vi "startIVSweepAndWait.vi"(8 "error in (no error)":errorcluster, 10 "setSweepConfiguration":variant, 11 "Instrument.LockinAPI in":refnum<class "Instrument.LockinAPI.lvclass">) -> (0 "error out":errorcluster, 3 "Instrument.LockinAPI out":refnum<class "Instrument.LockinAPI.lvclass">)   [LabVIEW 2019, in "Instrument.LockinAPI.lvclass"]
uses:
  Instrument.LockinAPI.lvclass
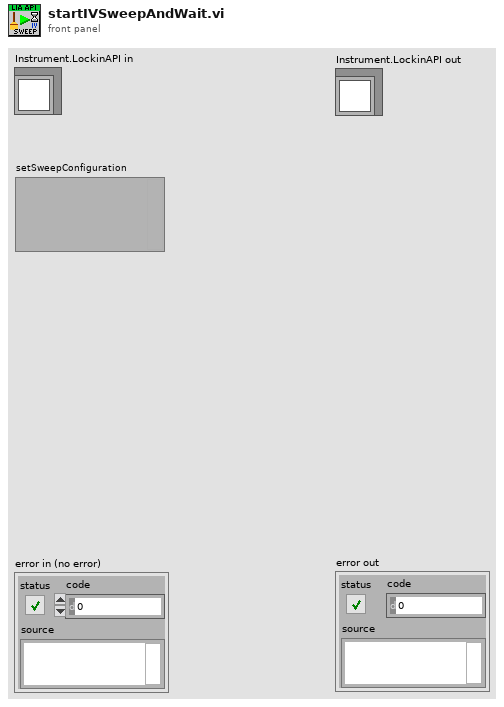
[diagram p1: front panel]
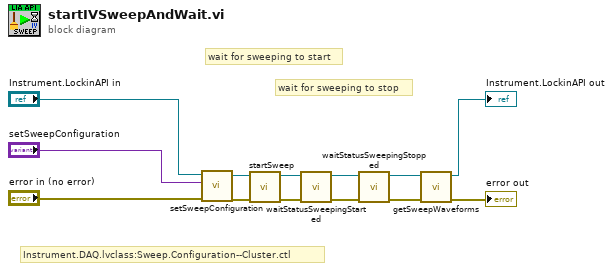
[diagram p0: block diagram]
diagram:
  # "Instrument.DAQ.lvclass:Sweep.Configuration--Cluster.ctl"
  # "wait for sweeping to stop"
  # "wait for sweeping to start"
  n1 = call-dynamic "setSweepConfiguration.vi"("error in (no error)"="error in (no error)", "setSweepConfiguration"="setSweepConfiguration", "Instrument.LockinAPI in"="Instrument.LockinAPI in") -> ("error out"=w9:errorcluster, "Instrument.LockinAPI out"=w10:refnum<class "Instrument.LockinAPI.lvclass">)  [unwired: 7 in]
  n2 = call "startSweep.vi"("error in (no error)"=w9, "Instrument.LockinAPI in"=w10) -> ("error out"=w5:errorcluster, "Instrument.LockinAPI out"=w6:refnum<class "Instrument.LockinAPI.lvclass">)  [unwired: 8 in]
  n3 = call "waitStatusSweepingStarted.vi"("error in (no error)"=w5, "Instrument.LockinAPI in"=w6) -> ("error out"=w4:errorcluster, "Instrument.LockinAPI out"=w7:refnum<class "Instrument.LockinAPI.lvclass">)  [unwired: 8 in]
  n4 = call "waitStatusSweepingStopped.vi"("error in (no error)"=w4, "Instrument.LockinAPI in"=w7) -> ("error out"=w3:errorcluster, "Instrument.LockinAPI out"=w2:refnum<class "Instrument.LockinAPI.lvclass">)  [unwired: 8 in]
  n5 = call-dynamic "getSweepWaveforms.vi"("error in (no error)"=w3, "Instrument.LockinAPI in"=w2) -> ("error out"=→"error out":errorcluster, "Instrument.LockinAPI out"=→"Instrument.LockinAPI out":refnum<class "Instrument.LockinAPI.lvclass">)  [unwired: 6 in, 2 out]
